vi "Create SUBSCRIBE Packet.vi"(5 "SUBSCRIBE in":refnum<class "SUBSCRIBE.lvclass">, 8 "error in (no error)":errorcluster, 9 "Packet ID (empty: Generate new)":u16 format="%04x", 11 "Topic Subscriptions":T1[](array[typedef])) -> (0 "error out":errorcluster, 2 "Bytes Stream":u8[](array[numeric]) format="%08b", 3 "SUBSCRIBE out":refnum<class "SUBSCRIBE.lvclass">)   [LabVIEW 2013, in "MQTT_Control_Packets.lvlib" / "SUBSCRIBE.lvclass"]
uses:
  SUBSCRIBE.lvclass
  Topic Subscription -- cluster.ctl
  ControlPacket/QualityOfService -- enum.ctl
  ControlPacket/ControlPacket.lvclass/ControlPacket.ctl
  ControlPacket/ControlPacket.lvclass
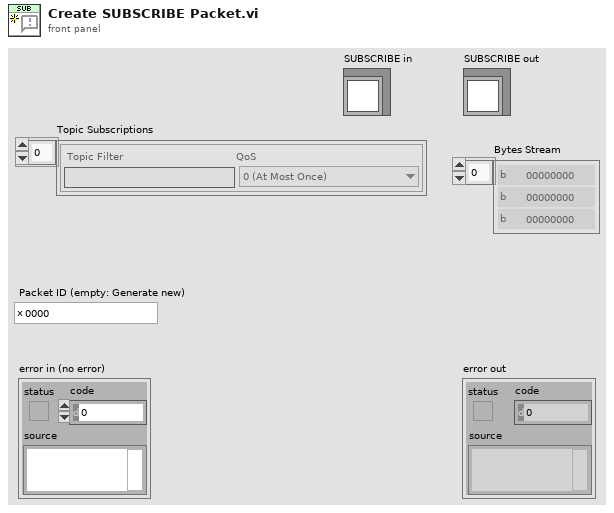
[diagram p1: front panel]
types:
  T1 = typedef "MQTT_Control_Packets.lvlib/SUBSCRIBE.lvclass/Topic Subscription -- cluster.ctl" = cluster{"Topic Filter":string, "QoS":T2}
  T2 = typedef "MQTT_Control_Packets.lvlib/ControlPacket.lvclass/QualityOfService -- enum.ctl" = enum16{"0 (At Most Once)", "1 (At Least Once)", "2 (Exactly Once)"}
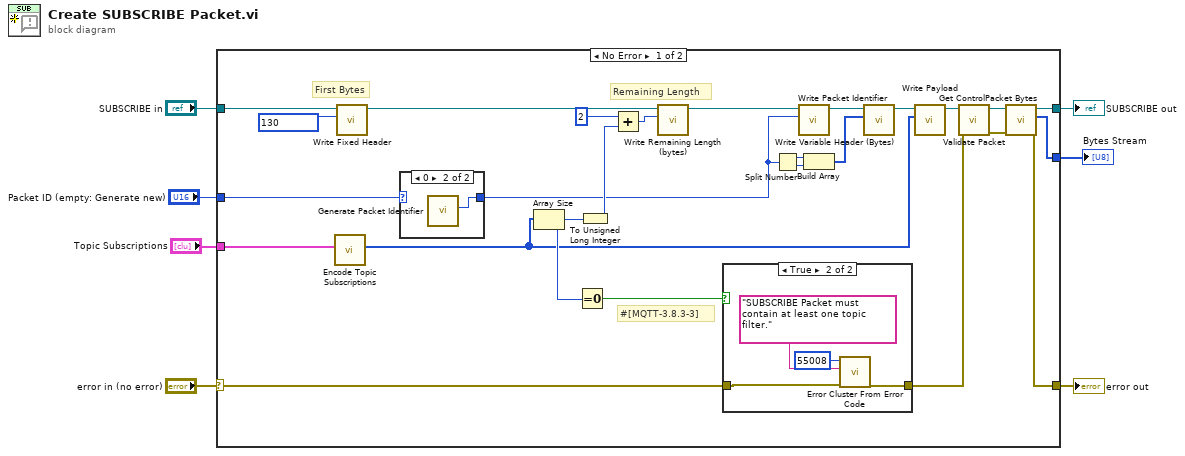
[diagram p0: block diagram]
diagram:
  n1 = case shown="No Error" "error in (no error)" {
    selector: "error in (no error)" -> [w20 w42]
    tunnel: [w8 w42] -> w4
    tunnel: [w11 w41] -> w3
    tunnel: "SUBSCRIBE in" -> [w33 w41]
    tunnel: "Packet ID (empty: Generate new)" -> [w13 _]
    tunnel: "Topic Subscriptions" -> [w18 _]
    tunnel: [w10 _] -> w1
    frame No Error {
      # "#[MQTT-3.8.3-3]"
      # "Remaining Length"
      # "First Bytes"
      n2 = call "Encode Topic Subscriptions.vi"("Topic Subscriptions"=w18) -> ("Payload"=w17:u8[])  [unwired: 10 in]
      n3 = call "Write Fixed Header.vi"("Fixed Header"=u8 130, "ControlPacket in"=w33) -> ("ControlPacket out"=w32:refnum<class "SUBSCRIBE.lvclass">)  [unwired: 9 in]
      n4 = case shown="0" w13 {
        selector: w13 -> [w34 _]
        tunnel: [w34 w35] -> w12
        frame Default {
        }
        frame 0 {
          n5 = call "Generate Packet Identifier.vi"() -> ("Packet Identifier"=w35:u16)  [unwired: 11 in]
        }
      }
      n6 = Array Size(array=w17) -> (size(s)=w21:i32)
      n7 = Equal To 0?(x=w21) -> (x = 0?=w19:bool)
      n8 = To Unsigned Long Integer(number=w21) -> (unsigned 32bit integer=w22:u32)
      n9 = Add(x=u32 2 ("Remaining Length (bytes)"), y=w22) -> (x+y=w24:u32)
      n10 = call "Write Remaining Length (bytes).vi"("Remaining Length (bytes)"=w24, "ControlPacket in"=w32) -> ("ControlPacket out"=w28:refnum<class "SUBSCRIBE.lvclass">)  [unwired: 9 in]
      n11 = case shown="True" w19 {
        tunnel: w20 -> [w36 w39]
        tunnel: [w36 w40] -> w16
        frame False {
        }
        frame True {
          n12 = call <vilib>:"Error Cluster From Error Code.vi"("error in (no error)"=w39, "error message (\"\")"="SUBSCRIBE Packet must contain at least one topic filter.", "error code (0)"=55008) -> ("error out"=w40:errorcluster)  [unwired: 6 in]
        }
      }
      n13 = Split Number(x=w12) -> (hi(x)=w31:u8, lo(x)=w30:u8)
      n14 = call "Write Packet Identifier.vi"("Packet Identifier"=w12, "ControlPacket in"=w28) -> ("ControlPacket out"=w27:refnum<class "SUBSCRIBE.lvclass">)  [unwired: 9 in]
      n15 = Build Array(w31, w30) -> (w29:u8[])
      n16 = call "Write Variable Header (Bytes).vi"("Variable Header (Bytes)"=w29, "ControlPacket in"=w27) -> ("ControlPacket out"=w23:refnum<class "SUBSCRIBE.lvclass">)  [unwired: 9 in]
      n17 = call "Write Payload.vi"("Payload"=w17, "ControlPacket in"=w23) -> ("ControlPacket out"=w14:refnum<class "SUBSCRIBE.lvclass">)  [unwired: 9 in]
      n18 = call "Validate Packet.vi"("error in (no error)"=w16, "ControlPacket in"=w14) -> ("error out"=w9:errorcluster, "ControlPacket out"=w15:refnum<class "SUBSCRIBE.lvclass">)  [unwired: 8 in]
      n19 = call "Get ControlPacket Bytes.vi"("error in (no error)"=w9, "ControlPacket"=w15) -> ("error out"=w8:errorcluster, "Bytes Stream"=w10:u8[], "ControlPacket dup"=w11:refnum<class "SUBSCRIBE.lvclass">)  [unwired: 6 in, 1 out]
    }
    frame Error {
    }
  }
  "error out" <- w4
  "SUBSCRIBE out" <- w3
  "Bytes Stream" <- w1
